vi "Enqueue One Command.vi"(8 "error in (no error)":errorcluster, 10 "Data":variant, 11 "Command":T1=enum."Shutdown Module") -> (0 "error out":errorcluster)   [LabVIEW 2022 SP3]
doc: "Issues a command by enqueuing into the module's command queue. The command should be received by calling the 'Dequeue' VI."
uses:
  Command.ctl
  Message.ctl
panel:
  # "Development\ncontrols/indicators useful for development and testing, but which are not outputs of the VI"
  # "Input\nInputs to the VI"
  # "Output\nOutputs of the VI"
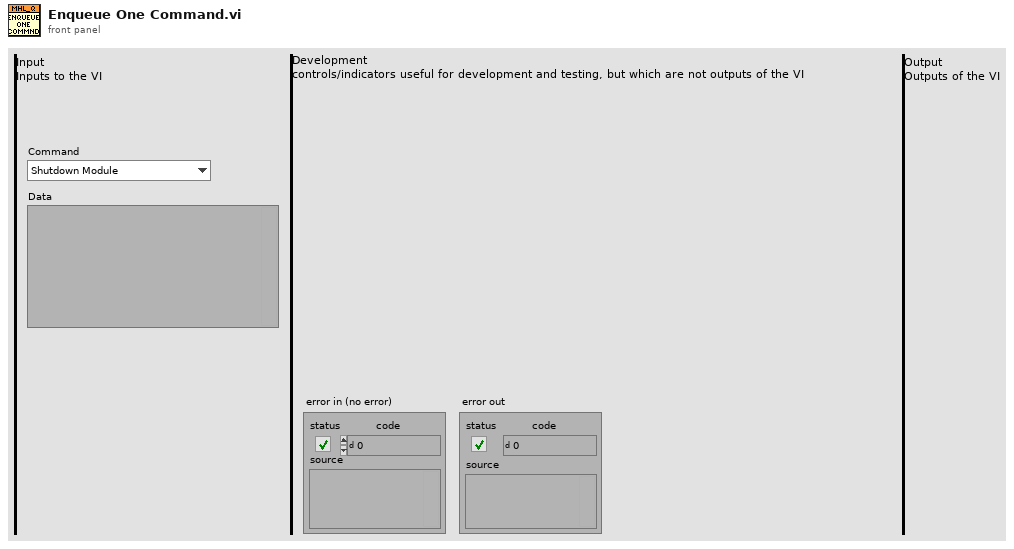
[diagram p1: front panel]
types:
  T1 = typedef "Command.ctl" = enum16{"Init Module", "Shutdown Module", "Local Error Handler", "Init Tickboxes", "Handle Value Change - Add to Project", "Handle Value Change - Add to Owner", "Handle Value Change - Add to Virtual Folder"}
  T2 = typedef "Message.ctl" = cluster{"Command":T1, "Data":variant}
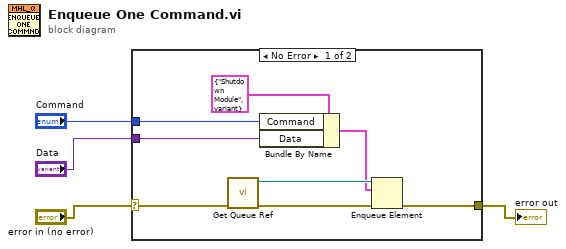
[diagram p0: block diagram]
diagram:
  n1 = case shown="No Error" "error in (no error)" {
    selector: "error in (no error)" -> [w12 w13]
    tunnel: [w10 w13] -> w3
    tunnel: "Command" -> [w6 _]
    tunnel: "Data" -> [w5 _]
    frame No Error {
      n2 = call "Get Queue Ref.vi"("error in (no error)"=w12) -> ("error out"=w11:errorcluster, "Queue Ref"=w9:refnum<queue>)  [unwired: 9 in]
      n3 = Bundle By Name(cluster=T2 {"Command"=enum."Shutdown Module", "Data"=variant} ("Queue Message"), "Command"=w6, "Data"=w5) -> (w7:T2)
      n4 = Enqueue Element(queue=w9, element=w7, error in (no error)=w11) -> (error out=w10:errorcluster)  [unwired: 1 in, 2 out]
    }
    frame Error {
    }
  }
  "error out" <- w3
